vi "Auto Broadcast State.vi"(5 "CSM Name":string, 8 "Current State":string, 9 "States Queue":string) -> (3 "Remaining States Queue":string)   [LabVIEW 2017, in "Communicable State Machine.lvlib"]
uses:
  Communicable State Machine.lvlib
  ChangeFlag/FlagInstance-CSMQ FGV.vi
  ChangeFlag/FlagInstance-Broadcast Cache.vi
  ChangeFlag/ChangeFlag-Read.vi
  FGV-BroadcastRegistry(lvlibp).vi
  AdvanceAPI/CSM - List Modules.vi
  _Shared/Trim Single-line Text.vi
  ChangeFlag/ChangeFlagDB.vi
  _Shared/CSM Shared.lvlib
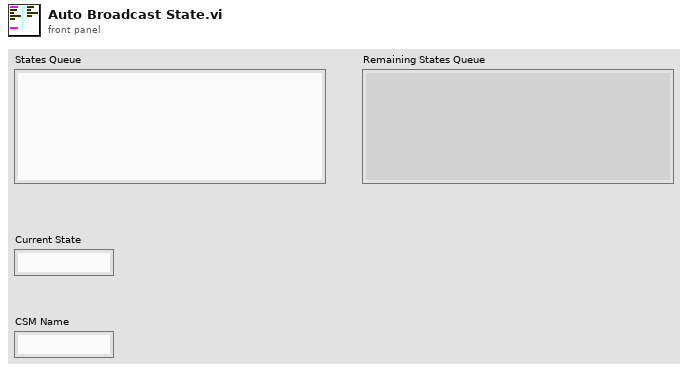
[diagram p1: front panel]
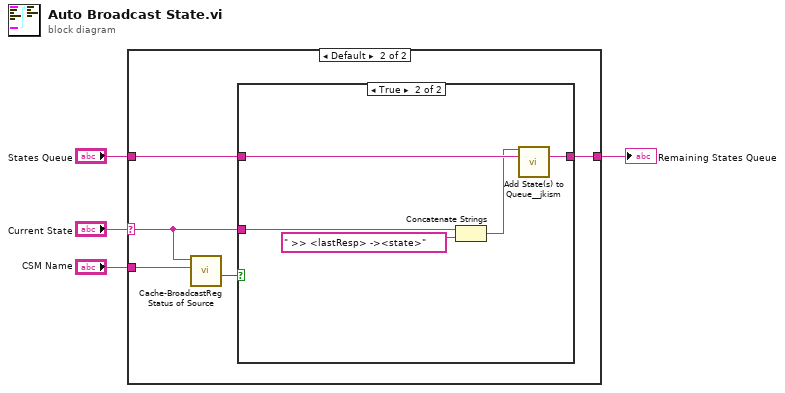
[diagram p0: block diagram]
diagram:
  n1 = case shown="Default" "Current State" {
    selector: "Current State" -> [_ w7]
    tunnel: [w5 w10] -> w3
    tunnel: "States Queue" -> [w5 w9]
    tunnel: "CSM Name" -> [_ w8]
    frame "" {
    }
    frame Default {
      n2 = call "Cache-BroadcastReg Status of Source.vi"("CSM Name"=w8, "Broadcast State"=w7) -> ("State Matched"=w6:bool)  [unwired: 8 in, 1 out]
      n3 = case shown="True" w6 {
        tunnel: w7 -> [_ w16]
        tunnel: [w11 w14] -> w10
        tunnel: w9 -> [w11 w13]
        frame False {
        }
        frame True {
          n4 = Concatenate Strings(w16, " >> <lastResp> -><state>" ("string")) -> (w12:string)
          n5 = call "Add State(s) to Queue__jkism.vi"("State(s) in Front (\"\")"=w12, "State(s) in (\"\")"=w13) -> ("States Out"=w14:string)  [unwired: 13 in]
        }
      }
    }
  }
  "Remaining States Queue" <- w3
